vi "Length Value Unit to Register Data.vi"(0 "Length Value":dbl=100.0 caption="长度值" min=0.0 format="%#.6g", 3 "Length Unit":u16(ring) caption="长度单位" items=["mm"]) -> (7 "Valid Result":bool caption="有效结果", 9 "Value Reg Data":dbl caption="值寄存器", 10 "Unit Reg Data":dbl caption="单位寄存器")   [LabVIEW 2023, in "Longer Pump dLSP501 Series.lvlib"]
uses:
  <instrlib>/Longer Pump dLSP501 Modbus RTU Series/Longer Pump dLSP501 Series.lvlib
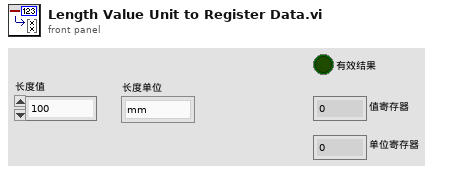
[diagram p1: front panel]
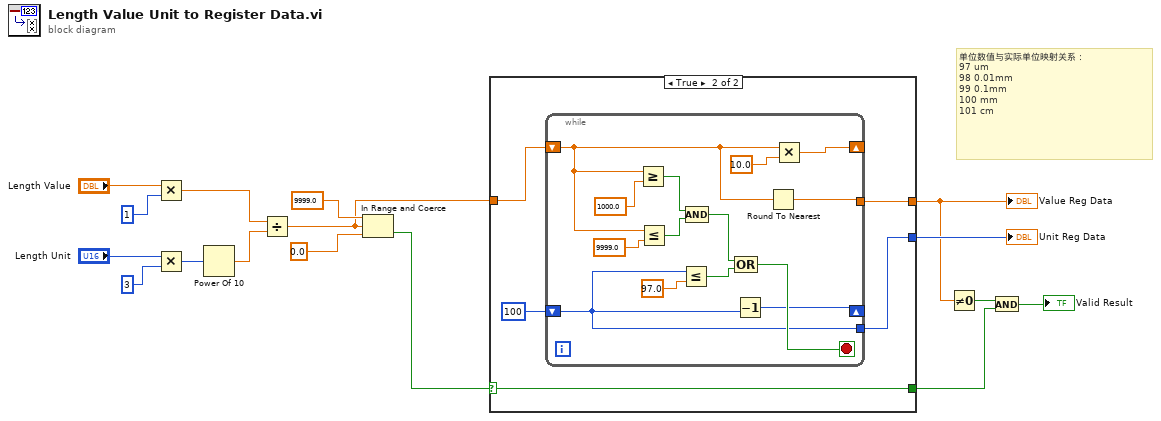
[diagram p0: block diagram]
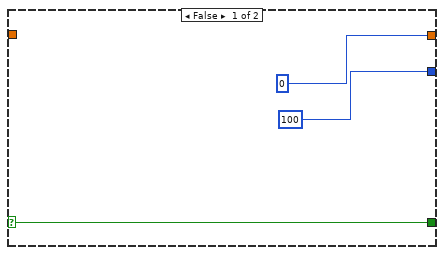
[diagram p2: hidden frame]
diagram:
  # "单位数值与实际单位映射关系：\n97\tum\n98\t0.01mm\n99\t0.1mm\n100\tmm\n101\tcm"
  n1 = Multiply(x="Length Value", y=u16 1) -> (x*y=w11:dbl)
  n2 = Multiply(x="Length Unit", y=u16 3) -> (x*y=w14:u16)
  n3 = Power Of 10(x=w14) -> (10^x=w10:dbl)
  n4 = Divide(x=w11, y=w10) -> (x/y=w6:dbl)
  n5 = In Range and Coerce(upper limit=9999.0 ("x"), x=w6, lower limit=0.0 ("x")) -> (In Range?=w7:bool)  [unwired: 1 out]
  n6 = case shown="True" w7 {
    selector: w7 -> [w19 w24]
    tunnel: w6 -> [_ w23]
    tunnel: [w19 w24] -> w1
    tunnel: [100 w20] -> w5
    tunnel: [0 w21] -> w3
    frame False {
    }
    frame True {
      n7 = while {
        shift-right: [w38] -> _
        shift-left: w23 -> [w26]
        shift-right: [w29] -> _
        shift-left: 100 -> [w27]
        tunnel: [w25] -> w21
        tunnel: [w27] -> w20
        stop <- w31 stop-if-true
        n8 = Greater Or Equal?(x=w26, y=1000.0 ("x")) -> (x >= y?=w34:bool)
        n9 = Less Or Equal?(x=w26, y=9999.0 ("x")) -> (x <= y?=w33:bool)
        n10 = Less Or Equal?(x=w27, y=97.0 ("x")) -> (x <= y?=w28:bool)
        n11 = Compound Arithmetic op=AND ("复合运算")(w34, w33) -> (w32:bool)
        n12 = Compound Arithmetic op=OR ("复合运算")(w32, w28) -> (w31:bool)
        n13 = Decrement(x=w27) -> (x-1=w29:i32)
        n14 = Round To Nearest(number=w26) -> (nearest integer value=w25:dbl)
        n15 = Multiply(x=w26, y=10.0) -> (x*y=w38:dbl)
      }
    }
  }
  "Value Reg Data" <- w3
  "Unit Reg Data" <- w5
  n16 = Not Equal To 0?(x=w3) -> (x != 0?=w4:bool)
  n17 = And(x=w4, y=w1) -> (x .and. y?=→"Valid Result":bool)
